vi "Lift.vi"(0 "Arm":bool, 1 "Winch":bool) -> ()   [LabVIEW 2018]
uses:
  <vilib>/Rock Robotics/WPI/Solenoid/WPI_SolenoidValue.ctl
  <vilib>/Rock Robotics/WPI/Solenoid/WPI_SolenoidSetEnum.vi
panel:
  in  "winchSpd":dbl=-0.5
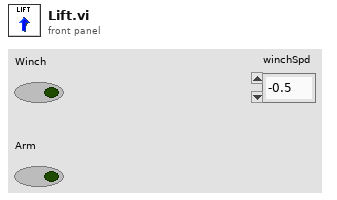
[diagram p1: front panel]
types:
  T1 = typedef "WPI_SolenoidValue.ctl" = enum16{"Off", "On", "Forward", "Reverse"}
  T2 = typedef "WPI_MotorControlDeviceRef.ctl" = cluster{"DeviceStatus":errorcluster, "Type":T3, "PWM":cluster{"PWM Channel":T4, "DeadBand":T5}, "CAN":cluster{"Device Number":u8, "SetOutput VI Ref":variant, "GetOutput VI Ref":variant, "Enable VI Ref":variant, "Disable VI Ref":variant, "Data":variant}, "Invert":bool, "DIO PWM":cluster{"PWM \"Enable\" Channel":T4, "DIOChannel":T6, "PWM Rate":dbl}}
  T3 = typedef "WPI_MotorControlType.ctl" = enum16{"PWM", "CAN", "DIO PWM"}
  T4 = typedef "FPGA_DIOPWMChannel.ctl" = enum8{"PWM 0", "PWM 1", "PWM 2", "PWM 3", "PWM 4", "PWM 5", "PWM 6", "PWM 7", "PWM 8", "PWM 9", "PWM MXP 0", "PWM MXP 1", "PWM MXP 2", "PWM MXP 3", "PWM MXP 4", "PWM MXP 5", "PWM MXP 6", "PWM MXP 7", "PWM MXP 8", "PWM MXP 9", "Invalid"}
  T5 = typedef "WPI_PWMDeadband.ctl" = cluster{"Name":string, "maxPositivePwm":i32, "minPositivePwm":i32, "centerPwm":i32, "maxNegativePwm":i32, "minNegativePwm":i32, "angularRange":u16}
  T6 = typedef "FPGA_DIOChannel.ctl" = enum8{"DIO 0", "DIO 1", "DIO 2", "DIO 3", "DIO 4", "DIO 5", "DIO 6", "DIO 7", "DIO 8", "DIO 9", "DIO MXP 0", "DIO MXP 1", "DIO MXP 2", "DIO MXP 3", "DIO MXP 4", "DIO MXP 5", "DIO MXP 6", "DIO MXP 7", "DIO MXP 8", "DIO MXP 9", "DIO MXP 10", "DIO MXP 11", "DIO MXP 12", "DIO MXP 13", "DIO MXP 14", "DIO MXP 15", "SPI Port CS1", "SPI Port CS2", "SPI Port CS3", "SPI Port MISO", "SPI Port MOSI", "Invalid"}
  T7 = typedef "WPI_SolenoidDevRef.ctl" = cluster{"DevStatus":errorcluster, "Pneumatics Control Module":u8, "Forward Solenoid Channel":T8, "Reverse Solenoid Channel":T8}
  T8 = typedef "WPI_SolenoidChannel.ctl" = enum8{"Solenoid 0", "Solenoid 1", "Solenoid 2", "Solenoid 3", "Solenoid 4", "Solenoid 5", "Solenoid 6", "Solenoid 7", "Invalid"}
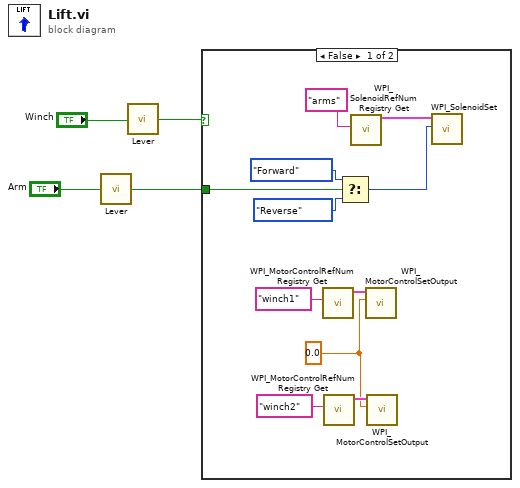
[diagram p0: block diagram]
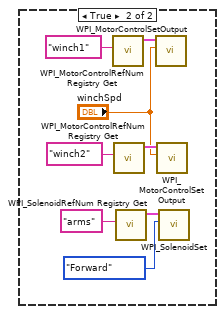
[diagram p2: hidden frame]
diagram:
  n1 = call "Lever.vi"("Input"="Arm") -> ("Output"=w1:bool)
  n2 = call "Lever.vi"("Input"="Winch") -> ("Output"=w2:bool)
  n3 = case shown="False" w2 {
    tunnel: w1 -> [w11 _]
    frame False {
      w5 = 0.0 ("Output")
      n4 = call <vilib>:"WPI_MotorControlRefNum Registry Get.vi"("refnum name"="winch1") -> ("MotorControlDevRef"=w9:T2)  [unwired: 9 in, 1 out]
      n5 = call <vilib>:"WPI_MotorControlRefNum Registry Get.vi"("refnum name"="winch2") -> ("MotorControlDevRef"=w7:T2)  [unwired: 9 in, 1 out]
      n6 = Select(t=WPI_SolenoidValue."Forward" ("Value"), s=w11, f=WPI_SolenoidValue."Reverse" ("Value")) -> (s? t:f=w10:T1)
      n7 = call <vilib>:"WPI_SolenoidRefNum Registry Get.vi"("refnum name"="arms") -> ("SolenoidDevRef"=w12:T7)  [unwired: 9 in, 1 out]
      n8 = call <vilib>:"WPI_MotorControlSetOutput.vi"("Output"=w5, "MotorControlDevRef"=w9) -> ()  [unwired: 7 in, 3 out]
      n9 = call <vilib>:"WPI_MotorControlSetOutput.vi"("Output"=w5, "MotorControlDevRef"=w7) -> ()  [unwired: 7 in, 3 out]
      n10 = call-poly <vilib>:"WPI_SolenoidSet.vi"("Value"=w10, "SolenoidDevRef"=w12) -> ()  [unwired: 8 in, 2 out]
    }
    frame True {
      n11 = call <vilib>:"WPI_MotorControlRefNum Registry Get.vi"("refnum name"="winch1") -> ("MotorControlDevRef"=w21:T2)  [unwired: 9 in, 1 out]
      n12 = call <vilib>:"WPI_MotorControlRefNum Registry Get.vi"("refnum name"="winch2") -> ("MotorControlDevRef"=w18:T2)  [unwired: 9 in, 1 out]
      n13 = call <vilib>:"WPI_SolenoidRefNum Registry Get.vi"("refnum name"="arms") -> ("SolenoidDevRef"=w23:T7)  [unwired: 9 in, 1 out]
      n14 = call <vilib>:"WPI_MotorControlSetOutput.vi"("Output"="winchSpd", "MotorControlDevRef"=w21) -> ()  [unwired: 7 in, 3 out]
      n15 = call <vilib>:"WPI_MotorControlSetOutput.vi"("Output"="winchSpd", "MotorControlDevRef"=w18) -> ()  [unwired: 7 in, 3 out]
      n16 = call-poly <vilib>:"WPI_SolenoidSet.vi"("Value"=WPI_SolenoidValue."Forward", "SolenoidDevRef"=w23) -> ()  [unwired: 8 in, 2 out]
    }
  }
